vi "Stop Core.vi"(10 "final error code":i32, 11 "Measurement in":refnum<class "Measurement.lvclass">) -> (3 "Measurement out":refnum<class "Measurement.lvclass">)   [LabVIEW 2015, in "Measurement Actor.lvlib" / "Measurement.lvclass"]
uses:
  Measurement.lvclass
  <vilib>/event_ctls.llb/usereventprio.ctl
  Measurement.lvclass/Measurement.ctl
  <vilib>/ActorFramework/Actor/Actor.lvclass
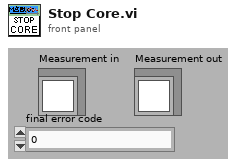
[diagram p1: front panel]
types:
  T1 = typedef "usereventprio.ctl" = enum32{"high priority", "normal priority"}
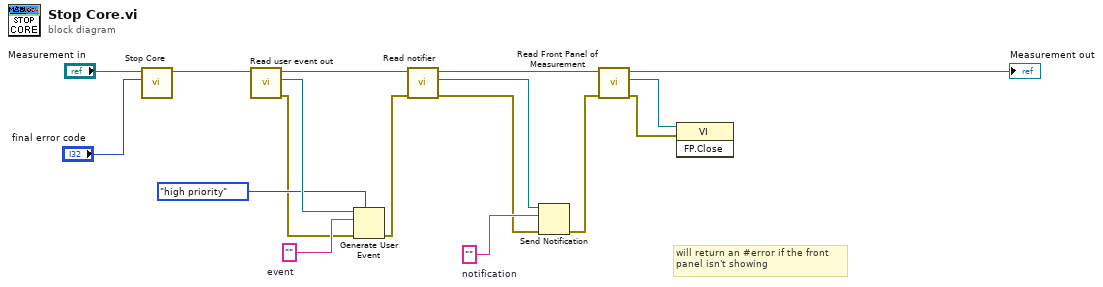
[diagram p0: block diagram]
diagram:
  w4 = ""  # event
  w15 = ""  # notification
  # "will return an #error if the front \npanel isn't showing"
  n1 = call-parent "Stop Core.vi"("final error code"="final error code", "Actor in"="Measurement in") -> ("Actor out"=w7:refnum<class "Measurement.lvclass">)  [unwired: 9 in]
  n2 = call "Read user event out.vi"("Measurement in"=w7) -> ("error out"=w3:errorcluster, "user event out"=w6:refnum<user-event>, "Measurement out"=w8:refnum<class "Measurement.lvclass">)  [unwired: 8 in]
  n3 = Generate User Event(priority (normal)=usereventprio."high priority", user event=w6, event data cluster=w4, error in=w3) -> (error out=w2:errorcluster)  [unwired: 1 out]
  n4 = call "Read notifier.vi"("error in (no error)"=w2, "Measurement in"=w8) -> ("error out"=w11:errorcluster, "notifier"=w16:refnum<notifier>, "Measurement out"=w12:refnum<class "Measurement.lvclass">)  [unwired: 7 in]
  n5 = Send Notification(notification=w15, notifier=w16, error in (no error)=w11) -> (error out=w10:errorcluster)  [unwired: 1 out]
  n6 = call "Read Front Panel of Measurement.vi"("error in (no error)"=w10, "Measurement in"=w12) -> ("error out"=w1:errorcluster, "Front Panel of Measurement"=w9:refnum<vi>, "Measurement out"=→"Measurement out":refnum<class "Measurement.lvclass">)  [unwired: 7 in]
  n7 = invoke class="VI" method="FP.Close"(reference=w9, error in=w1) -> ()  [unwired: 1 in, 3 out]
